vi "Stacked Bar Waveform Graph.vi"() -> ()   [LabVIEW 2018]
doc: "This VI shows how to visualize data using a stacked graph. The stack plot is drawn using a waveform graph."
panel:
  in  "Raw Data":string[][](table)=[["3", "4", "1", "6", "2"], ["33", "26", "12", "100", "23"], ["4", "3", "1", "8", "2"], ["4", "8", "4", "12", "4"], ["2", "3", "1", "9", "3"], ["3", "2", "3", "12", "1"]]
  out "Stacked Bar Plots":dbl[][](graph)
  # "Overview: Illustrates the use of the waveform graph to display stacked bar plots.\nInstructions:\nRun the VI."
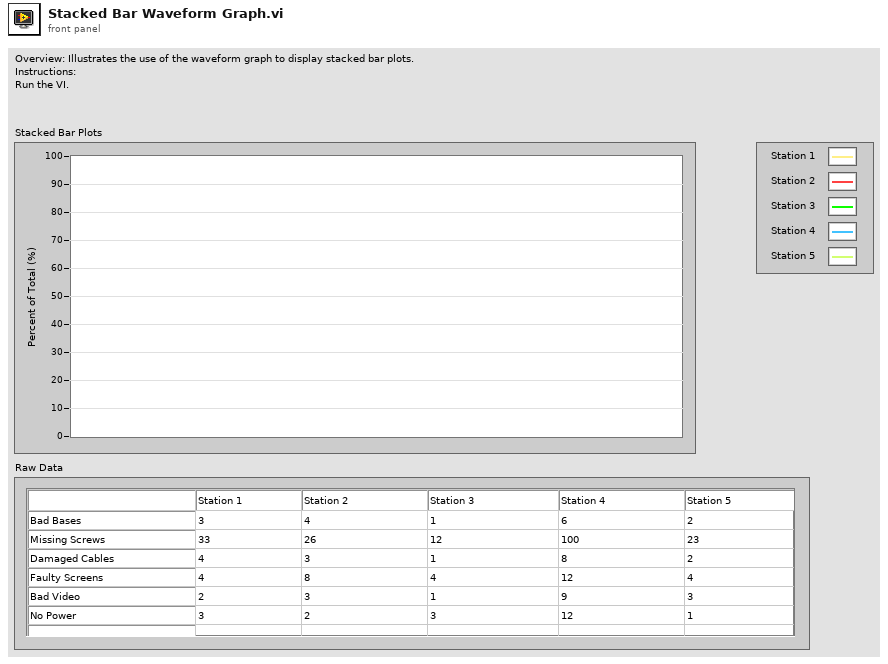
[diagram p1: front panel]
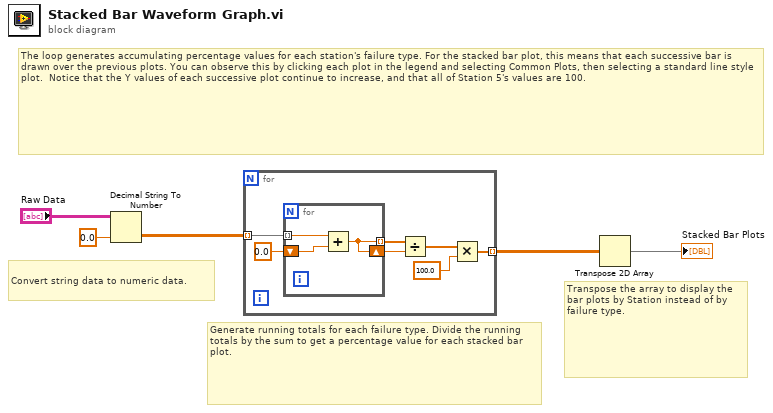
[diagram p0: block diagram]
diagram:
  # "The loop generates accumulating percentage values for each station's failure type. For the stacked bar plot, this means that each successive bar is drawn over the previous plots. You can observe this by clicking each plot in the legend and selecting Common Plots, then selecting a standard line style plot.  Notice that the Y values of each successive plot continue to increase, and that all of Station 5's values are 100."
  # "Generate running totals for each failure type. Divide the running totals by the sum to get a percentage value for each stacked bar plot."
  # "Transpose the array to display the bar plots by Station instead of by failure type."
  # "Convert string data to numeric data."
  n1 = Decimal String To Number(string="Raw Data", default (0L)=0.0) -> (number=w4:dbl[][])  [unwired: 1 in, 1 out]
  n2 = for {
    tunnel: w4 -> [w12] mode=indexing
    tunnel: [w10] -> w5 mode=indexing
    n3 = for {
      shift-right: [w14] -> w9
      shift-left: 0.0 -> [w13]
      tunnel: w12 -> [w15] mode=indexing
      tunnel: [w14] -> w11 mode=indexing
      n4 = Add(x=w15, y=w13) -> (x+y=w14:dbl)
    }
    n5 = Divide(x=w11, y=w9) -> (x/y=w8:dbl[])
    n6 = Multiply(x=w8, y=100.0) -> (x*y=w10:dbl[])
  }
  n7 = Transpose 2D Array(2D array=w5) -> (transposed array=→"Stacked Bar Plots":dbl[][])
